vi "scan - Copy.vi"(8 "error in (no error)":errorcluster, 11 "Input":string="0,-110n,10n,64") -> (0 "error out":errorcluster, 3 "Output":string)   [LabVIEW 2014]
uses:
  <userlib>/Nanonis Prog Interface V5/Nanonis Prog Interface.lvlib
panel:
  in  "min distance for creep":dbl
  in  "seconds to wait":dbl=3.0
  in  "Angle (deg)":sgl=nan caption="Angle (deg) (NaN=no change)" format="%.2f"
  in  "Size (m)":cluster{"Width":sgl, "Height":sgl}={"Width"=1e-08, "Height"=1e-08} caption="Size (m) (NaN=no change)" {"Height" format="%.2p"; "Width" format="%.2p"}
  out "size(s)":i32=4
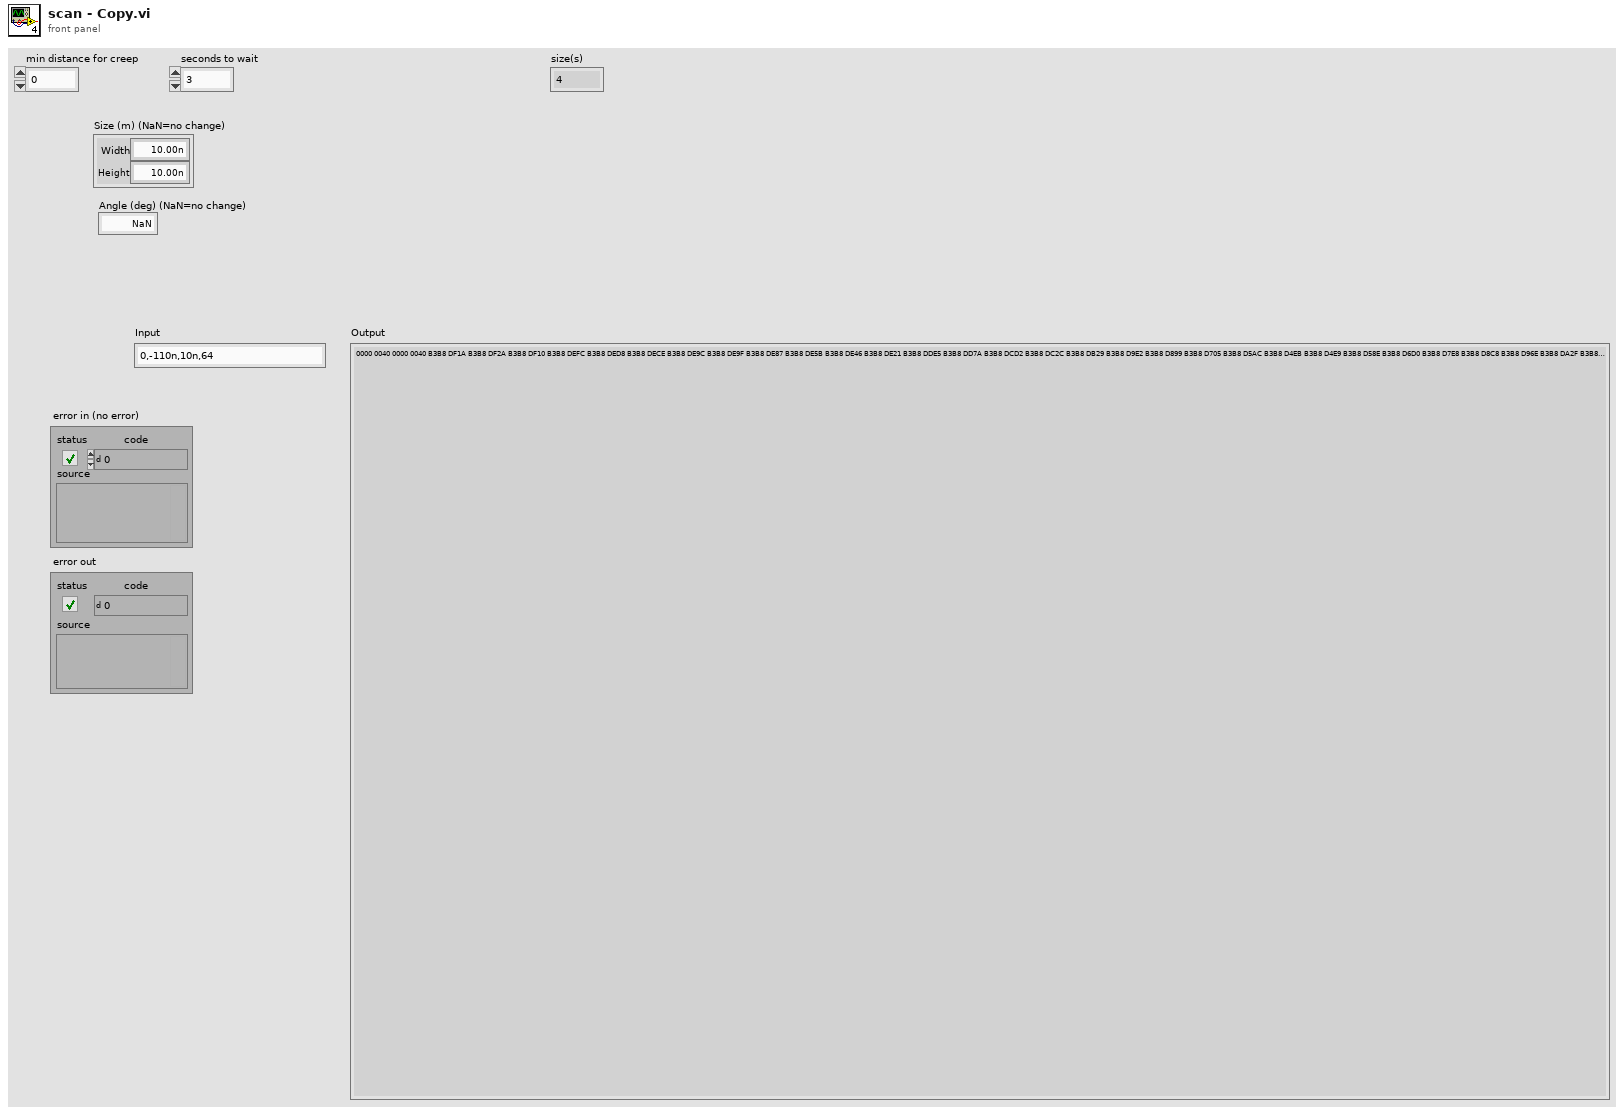
[diagram p1: front panel]
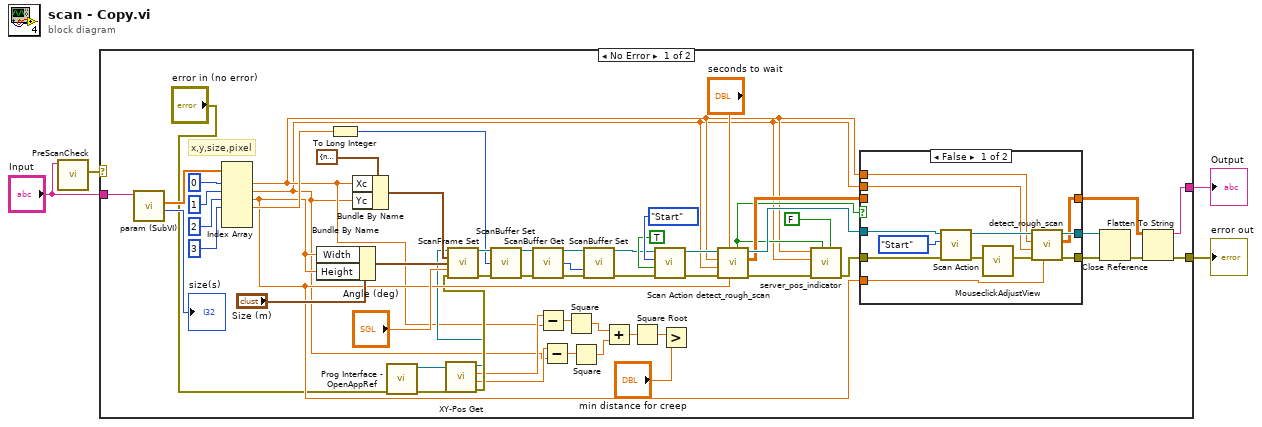
[diagram p0: block diagram]
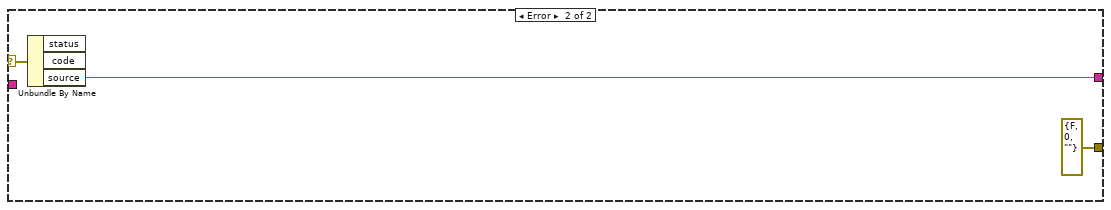
[diagram p3: hidden frame]
diagram:
  n1 = call "PreScanCheck.vi"("Input"="Input") -> ("error"=w1:errorcluster)  [unwired: 8 in, 2 out]
  n2 = case shown="No Error" w1 {
    selector: w1 -> [_ w78]
    tunnel: [w44 w77] -> w4
    tunnel: [w36 errorcluster {"status"=FALSE, "code"=0, "source"=""} ("error out")] -> w3
    tunnel: "Input" -> [w33 _]
    frame No Error {
      # "x,y,size,pixel"
      n3 = call <userlib>:"param (SubVI).vi"("Input"=w33) -> ("num"=→"size(s)":i32, "parm"=w60:dbl[])  [unwired: 8 in, 1 out]
      n4 = Index Array(array=w60, index #1=0 ("index"), index #2=1 ("index"), index #3=2 ("index"), index #4=3 ("index")) -> (element #1=w13:dbl, element #2=w12:dbl, element #3=w24:dbl, element #4=w46:dbl)  [unwired: 2 in, 2 out]
      n5 = Bundle By Name(cluster="Size (m)", "Width"=w24, "Height"=w24) -> (w47:cluster{"Width":sgl, "Height":sgl})
      n6 = To Long Integer(number=w46) -> (32bit integer=w45:i32)
      n7 = Bundle By Name(cluster=cluster{"Xc":sgl, "Yc":sgl} {"Xc"=nan, "Yc"=nan} ("Center coordinates (m)"), "Xc"=w13, "Yc"=w12) -> (w58:cluster{"Xc":sgl, "Yc":sgl})
      n8 = call <userlib>:"Prog Interface - OpenAppRef.vi"("Error in (no error)"="error in (no error)") -> ("Error out"=w19:errorcluster, "Application reference"=w18:refnum<vi>)  [unwired: 5 in]
      n9 = call <userlib>:"XY-Pos Get.vi"("error in (no error)"=w19, "Application ref in"=w18) -> ("error out"=w17:errorcluster, "Y (m)"=w14:sgl, "X (m)"=w15:sgl, "Application ref out"=w16:refnum<vi>)  [unwired: 5 in]
      n10 = call <userlib>:"ScanFrame Set.vi"("Application ref in"=w16, "Center coordinates (m)"=w58, "Size (m)"=w47, "Angle (deg)"="Angle (deg)", "error in (no error)"=w17) -> ("Application ref out"=w56:refnum<vi>, "error out"=w55:errorcluster)  [unwired: 9 in]
      n11 = call <userlib>:"ScanBuffer Set.vi"("Application ref in"=w56, "Pixels"=w45, "error in (no error)"=w55) -> ("Application ref out"=w40:refnum<vi>, "error out"=w39:errorcluster)  [unwired: 11 in]
      n12 = call <userlib>:"ScanBuffer Get.vi"("Application ref in"=w40, "error in (no error)"=w39) -> ("Application ref out"=w42:refnum<vi>, "Pixels/line"=w43:i32, "error out"=w41:errorcluster)  [unwired: 9 in, 2 out]
      n13 = Subtract(x=w15, y=w13) -> (x-y=w11:dbl)
      n14 = Subtract(x=w14, y=w12) -> (x-y=w10:dbl)
      n15 = Square(x=w11) -> (x^2=w9:dbl)
      n16 = Square(x=w10) -> (x^2=w8:dbl)
      n17 = call <userlib>:"ScanBuffer Set.vi"("Application ref in"=w42, "Lines"=w43, "error in (no error)"=w41) -> ("Application ref out"=w38:refnum<vi>, "error out"=w37:errorcluster)  [unwired: 11 in]
      n18 = Add(x=w9, y=w8) -> (x+y=w7:dbl)
      n19 = Square Root(x=w7) -> (sqrt(x)=w6:dbl)
      n20 = call <userlib>:"Scan Action.vi"("error in (no error)"=w37, "Direction: up/down (T=up)"=TRUE, "Scan action (Start)"=enum16{"Start", "Stop", "Pause", "Resume"}."Start", "Application ref in"=w38) -> ("error out"=w27:errorcluster, "Application ref out"=w28:refnum<vi>)  [unwired: 5 in]
      n21 = Greater?(x=w6, y="min distance for creep") -> ()  [unwired: 1 out]
      n22 = call "detect_rough_scan.vi"("size (m)"=w24, "max scan time"="seconds to wait", "Error in"=w27, "Y (m)"=w12, "X (m)"=w13, "App in"=w28) -> ("error out"=w23:errorcluster, "Array"=w25:sgl[][], "Application ref out"=w26:refnum<vi>, "rough image detected"=w21:bool)  [unwired: 2 in]
      n23 = call "server_pos_indicator.vi"("reset"=FALSE, "rough"=w21, "error in"=w23, "yc"=w12, "xc"=w13) -> ("error out"=w22:errorcluster)  [unwired: 6 in]
      n24 = case shown="False" w21 {
        tunnel: [w73 w75] -> w32
        tunnel: [w72 w74] -> w31
        tunnel: [w69 w76] -> w30
        tunnel: w26 -> [w66 w75]
        tunnel: w22 -> [w65 w74]
        tunnel: w25 -> [_ w76]
        tunnel: w13 -> [w64 _]
        tunnel: w12 -> [w63 _]
        tunnel: w24 -> [w62 _]
        frame False {
          n25 = call <userlib>:"Scan Action.vi"("error in (no error)"=w65, "Scan action (Start)"=enum16{"Start", "Stop", "Pause", "Resume"}."Start", "Application ref in"=w66) -> ("error out"=w67:errorcluster, "Application ref out"=w71:refnum<vi>)  [unwired: 6 in]
          n26 = call "MouseclickAdjustView.vi"("error in (no error)"=w67) -> ("error out"=w70:errorcluster)  [unwired: 10 in]
          n27 = call "detect_rough_scan.vi"("size (m)"=w62, "Error in"=w70, "Y (m)"=w63, "X (m)"=w64, "App in"=w71) -> ("error out"=w72:errorcluster, "Array"=w69:sgl[][], "Application ref out"=w73:refnum<vi>)  [unwired: 3 in, 1 out]
        }
        frame True {
        }
      }
      n28 = Close Reference(reference=w32, error in (no error)=w31) -> (error out=w34:errorcluster)
      n29 = Flatten To String(anything=w30, error in (no error)=w34) -> (data string=w44:string, error out=w36:errorcluster)  [unwired: 2 in, 1 out]
    }
    frame Error {
      n30 = Unbundle By Name(w78) -> ("source"=w77:string)  [unwired: 2 out]
    }
  }
  "Output" <- w4
  "error out" <- w3
